vi "Compile Status Channels FIFO Indices.vi"(8 "error in (no error)":errorcluster, 11 "Device Ref in":T2 format="%.0x") -> (0 "error out":errorcluster, 2 "Status Channels FIFO Indices":T1, 3 "Device Ref out":T2 format="%.0x")   [LabVIEW 2020, in "Routing and Faulting System Explorer.lvlib"]
uses:
  Routing and Faulting System Explorer.lvlib
  <vilib>/NI VeriStand/Custom Device API/Custom Device Item Ref.ctl
  Shared/FIFO Indices.ctl
  Shared/Constants.vi
  <vilib>/NI VeriStand/Custom Device Tools/Custom Device Utility Library/Custom Device Utility Library.lvlib
  <vilib>/NI VeriStand/Custom Device API/Custom Device API.lvlib
  Shared/Routing and Faulting Shared.lvlib
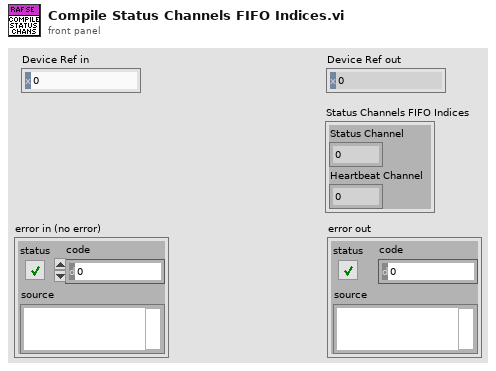
[diagram p1: front panel]
types:
  T1 = typedef "Routing and Faulting Shared.lvlib/FIFO Indices.ctl" = cluster{"Status Channel":i32, "Heartbeat Channel":i32}
  T2 = typedef "Custom Device API.lvlib/Custom Device Item Ref.ctl" = u64
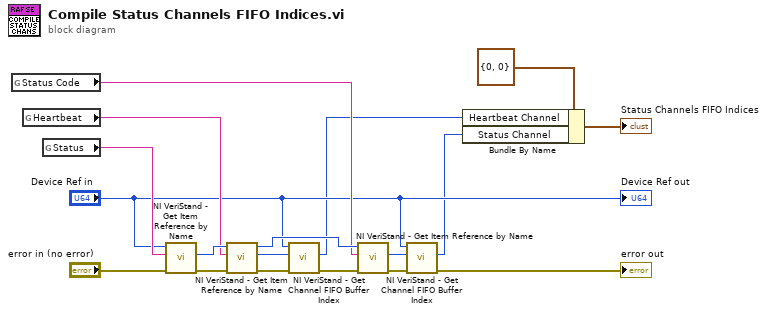
[diagram p0: block diagram]
diagram:
  n1 = global read "Constants.vi" "Status Code"() -> (w6:string)
  n2 = global read "Constants.vi" "Heartbeat"() -> (w7:string)
  n3 = global read "Constants.vi" "Status"() -> (w8:string)
  n4 = call <vilib>:"NI VeriStand - Get Item Reference by Name.vi"("error in (no error)"="error in (no error)", "Item Name"=w8, "Parent Ref in"="Device Ref in") -> ("error out"=w18:errorcluster, "Item Ref"=w17:T2)  [unwired: 5 in, 2 out]
  n5 = call <vilib>:"NI VeriStand - Get Item Reference by Name.vi"("error in (no error)"=w18, "Item Name"=w7, "Parent Ref in"=w17) -> ("error out"=w16:errorcluster, "Item Ref"=w15:T2, "Parent Ref out"=w13:T2)  [unwired: 5 in, 1 out]
  n6 = call <vilib>:"NI VeriStand - Get Channel FIFO Buffer Index.vi"("error in"=w16, "Channel Ref"=w15, "Device Ref in"="Device Ref in") -> ("error out"=w14:errorcluster, "Channel FIFO Buffer Index"=w3:i32)  [unwired: 4 in, 3 out]
  n7 = call <vilib>:"NI VeriStand - Get Item Reference by Name.vi"("error in (no error)"=w14, "Item Name"=w6, "Parent Ref in"=w13) -> ("error out"=w12:errorcluster, "Item Ref"=w11:T2)  [unwired: 5 in, 2 out]
  n8 = call <vilib>:"NI VeriStand - Get Channel FIFO Buffer Index.vi"("error in"=w12, "Channel Ref"=w11, "Device Ref in"="Device Ref in") -> ("error out"=→"error out":errorcluster, "Channel FIFO Buffer Index"=w2:i32)  [unwired: 4 in, 3 out]
  n9 = Bundle By Name(cluster=T1 {"Status Channel"=0, "Heartbeat Channel"=0} ("FIFO Indices"), "Heartbeat Channel"=w3, "Status Channel"=w2) -> (→"Status Channels FIFO Indices":T1)
  "Device Ref out" <- "Device Ref in"
